vi "X1 minus X0.vi"(7 "Reinit":bool, 8 "error in (no error)":errorcluster, 9 "X0":dbl, 10 "X1":dbl, 11 "Stats_DBL_CIF_U in":refnum<class "Stats_DBL_CIF_U.lvclass">) -> (0 "error out":errorcluster, 3 "Stats_DBL_CIF_U out":refnum<class "Stats_DBL_CIF_U.lvclass">)   [LabVIEW 2021, in "Stats_CIF_U.lvlib" / "Stats_DBL_CIF_U.lvclass"]
doc: "Load a new data value into the statistics class. The new value will be calculated by subracting the X value from the Y value. This VI is useful for benchmarking where a timestamp is taken before and after a function."
uses:
  Stats_DBL_CIF_U.lvclass
  Stats_DBL_CIF_U.lvclass/Stats_DBL_CIF_U.ctl
  dfabcf33-0dbc-4041-80a5-3dc0c86d2989.vi
  dfabcf33-0dbc-4041-80a5-3dc0c86d2989.vi/9eb60a9a-770f-4d2d-8b3f-8465c267ecc9.vi
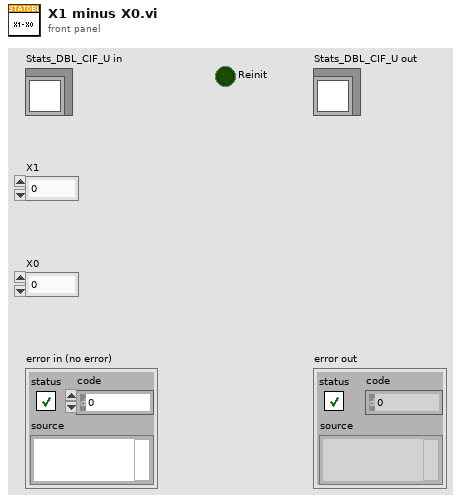
[diagram p1: front panel]
types:
  T1 = typedef "Stats_CIF_U.lvlib/DBL Stat Data.ctl" = cluster{"Last Value":dbl, "Max":dbl, "Min":dbl, "Common ":T2}
  T2 = typedef "Stats_CIF_U.lvlib/Common Stat Data.ctl" = cluster{"Iteration":u32, "Max History":i32, "Average":dbl, "Init":bool}
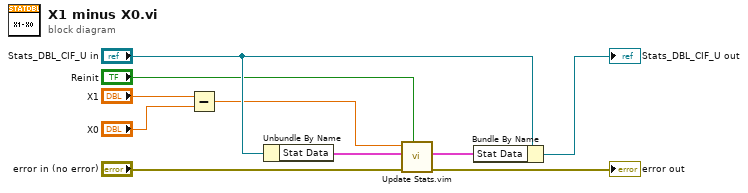
[diagram p0: block diagram]
diagram:
  n1 = Subtract(x="X1", y="X0") -> (x-y=w1:dbl)
  n2 = Unbundle By Name("Stats_DBL_CIF_U in") -> ("Stat Data"=w8:T1)
  n3 = call "Update Stats.vim"("Reinit"="Reinit", "error in"="error in (no error)", "Stat Data In"=w8, "New Value"=w1) -> ("error out"=→"error out":errorcluster, "Stat Data Out"=w7:T1)  [unwired: 6 in]
  n4 = Bundle By Name(cluster="Stats_DBL_CIF_U in", "Stat Data"=w7) -> (→"Stats_DBL_CIF_U out":refnum<class "Stats_DBL_CIF_U.lvclass">)
